vi "FM_Demodulator.vi"(1 "Array in":cdb[](array[numeric])) -> (0 "Array out":dbl[](array[numeric]))   [LabVIEW 2020]
uses:
  <vilib>/Analysis/NI_AAL_Angle.lvlib
  <vilib>/Analysis/coordinate.llb/Wrap Angle (scalar).vi
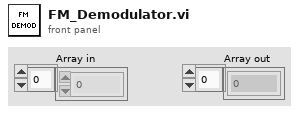
[diagram p1: front panel]
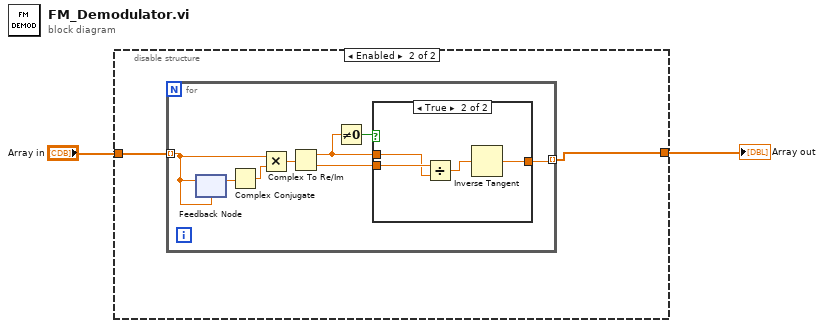
[diagram p0: block diagram]
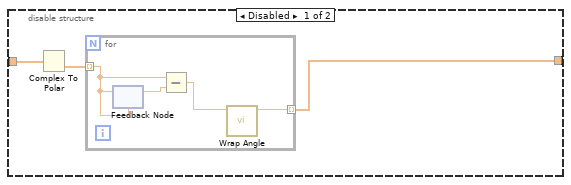
[diagram p2: hidden frame]
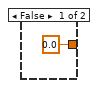
[diagram p3: hidden frame]
diagram:
  n1 = disable-structure shown="Enabled" {
    disable-tunnel: "Array in" -> [w5 w11]
    disable-tunnel: [w4 w10] -> w1
    frame Disabled {
      n2 = Complex To Polar(r * e^(i*theta)=w5) -> (theta=w3:dbl[])  [unwired: 1 out]
      n3 = for {
        tunnel: w3 -> [w6] mode=indexing
        tunnel: [w7] -> w4 mode=indexing
        n4 = feedback-in #1(w6) -> ()
        n5 = feedback #1(w6) -> (w9:dbl)
        n6 = Subtract(x=w6, y=w9) -> (x-y=w8:dbl)
        n7 = call-poly <vilib>:"Wrap Angle.vi"("angle in"=w8) -> ("angle out"=w7:dbl)  [unwired: 9 in, 1 out]
      }
    }
    frame Enabled {
      n8 = for {
        tunnel: w11 -> [w12] mode=indexing
        tunnel: [w19] -> w10 mode=indexing
        n9 = feedback-in #2(w12) -> ()
        n10 = feedback #2(w12) -> (w18:cdb)
        n11 = Complex Conjugate(1:w18) -> (0:w17:cdb)
        n12 = Multiply(x=w12, y=w17) -> (x*y=w16:cdb)
        n13 = Complex To Re/Im(x + iy=w16) -> (x=w13:dbl, y=w15:dbl)
        n14 = Not Equal To 0?(x=w13) -> (x != 0?=w14:bool)
        n15 = case shown="True" w14 {
          tunnel: [0.0 w24] -> w19
          tunnel: w15 -> [_ w23]
          tunnel: w13 -> [_ w22]
          frame False {
          }
          frame True {
            n16 = Divide(x=w23, y=w22) -> (x/y=w21:dbl)
            n17 = Inverse Tangent(1:w21) -> (0:w24:dbl)
          }
        }
      }
    }
  }
  "Array out" <- w1
